vi "Print XML Recursive Priv.vi"(0 "Tree Dictionary In":variant, 2 "Data Types Dict":variant, 7 "Child IDs":string[](array[string]), 11 "error in":errorcluster, 13 "Indent":i32) -> (4 "Tree Dictionary Out":variant, 8 "XML Lines":string[](array[string]), 15 "error out":errorcluster)   [LabVIEW 2017, in "Tree API.lvlib" / "Tree.lvclass"]
uses:
  Tree.lvclass
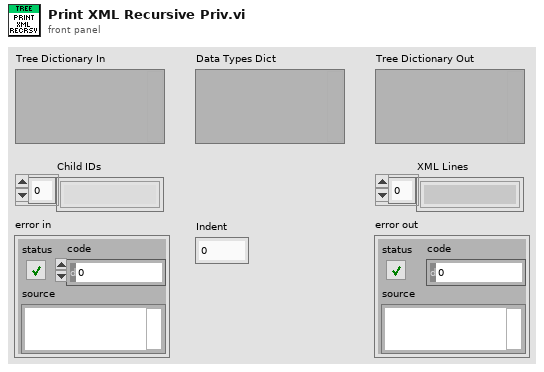
[diagram p1: front panel]
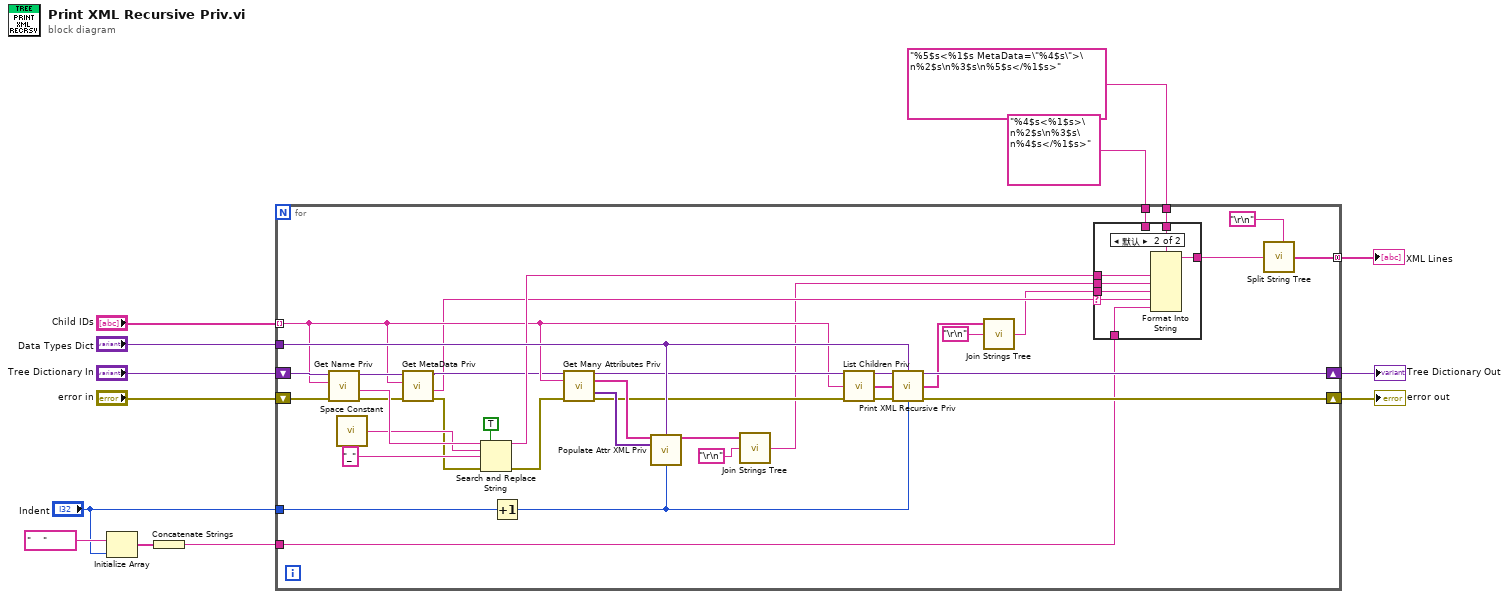
[diagram p0: block diagram]
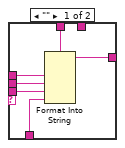
[diagram p2: hidden frame]
diagram:
  n1 = Initialize Array("    ", "Indent") -> (w3:string[])
  n2 = Concatenate Strings(w3) -> (w2:string)
  n3 = for {
    tunnel: "Child IDs" -> [w31] mode=indexing
    shift-right: [w48] -> w10
    shift-left: "Tree Dictionary In" -> [w51]
    shift-right: [w37] -> w13
    shift-left: "error in" -> [w50]
    tunnel: "Data Types Dict" -> [w46]
    tunnel: [w19] -> w1 mode=concatenating
    tunnel: "%5$s<%1$s MetaData=\"%4$s\">\n%2$s\n%3$s\n%5$s</%1$s>" ("format string") -> [w27]
    tunnel: "%4$s<%1$s>\n%2$s\n%3$s\n%4$s</%1$s>" ("format string") -> [w26]
    tunnel: "Indent" -> [w15]
    tunnel: w2 -> [w16]
    n4 = call "Get Name Priv.vi"("error in"=w50, "Unique ID"=w31, "Tree Dictionary"=w51) -> ("error out"=w32:errorcluster, "Name"=w43:string, "Tree Dictionary Out"=w33:variant)  [unwired: 6 in]
    n5 = call <vilib>:"Space Constant.vi"() -> ("String"=w42:string)
    n6 = call "Get MetaData Priv.vi"("error in"=w32, "Unique ID"=w31, "Tree Dictionary"=w33) -> ("error out"=w29:errorcluster, "MetaData"=w28:string, "Tree Dictionary Out"=w30:variant)  [unwired: 6 in]
    n7 = Search and Replace String(replace all?=TRUE ("replace all? (F)"), input string=w43, search string=w42, replace string="_", error in=w29) -> (result string=w39:string, error out=w38:errorcluster)  [unwired: 3 in, 2 out]
    n8 = Increment(x=w15) -> (x+1=w14:i32)
    n9 = call "Get Many Attributes Priv.vi"("Tree Dictionary In"=w30, "Unique ID"=w31, "error in"=w38) -> ("Tree Dictionary Out"=w44:variant, "Attribute Names"=w36:string[], "Attribute Values"=w35:variant[], "error out"=w34:errorcluster)  [unwired: 7 in, 2 out]
    n10 = call "Populate Attr XML Priv.vi"("Attribute Names"=w36, "Data Types Dict"=w46, "Attribute Values"=w35, "Indent"=w14) -> ("Attr XML Strings"=w18:string[])  [unwired: 11 in]
    n11 = call "Join Strings Tree.vi"("Separator (,)"="\r\n", "Strings In"=w18) -> ("String"=w22:string)  [unwired: 1 in]
    n12 = call "List Children Priv.vi"("Tree Dictionary"=w44, "Parent ID"=w31, "Error In"=w34) -> ("Tree Dictionary Out"=w49:variant, "Child IDs"=w47:string[], "Error Out"=w45:errorcluster)  [unwired: 10 in]
    n13 = call "Print XML Recursive Priv.vi"("Tree Dictionary In"=w49, "Data Types Dict"=w46, "Child IDs"=w47, "error in"=w45, "Indent"=w14) -> ("Tree Dictionary Out"=w48:variant, "XML Lines"=w17:string[], "error out"=w37:errorcluster)  [unwired: 8 in]
    n14 = call "Join Strings Tree.vi"("Separator (,)"="\r\n", "Strings In"=w17) -> ("String"=w24:string)  [unwired: 1 in]
    n15 = case shown="默认" w28 {
      selector: w28 -> [_ w60]
      tunnel: [w53 w64] -> w20
      tunnel: w24 -> [w55 w63]
      tunnel: w22 -> [w56 w62]
      tunnel: w39 -> [w57 w61]
      tunnel: w27 -> [_ w59]
      tunnel: w26 -> [w54 _]
      tunnel: w16 -> [w52 w58]
      frame "" {
        n16 = Format Into String(format string=w54, w57, w56, w55, w52) -> (resulting string=w53:string)  [unwired: 2 in, 1 out]
      }
      frame Default {
        n17 = Format Into String(format string=w59, w61, w62, w63, w60, w58) -> (resulting string=w64:string)  [unwired: 2 in, 1 out]
      }
    }
    n18 = call "Split String Tree.vi"("Split Pattern"="\r\n", "Input String"=w20) -> ("Split String"=w19:string[])  [unwired: 5 in]
  }
  "error out" <- w13
  "Tree Dictionary Out" <- w10
  "XML Lines" <- w1
